vi "Generate String.vi"(8 "error in (no error)":errorcluster, 11 "object in":refnum<class "RawCodeElement.lvclass">) -> (0 "error out":errorcluster, 2 "String":string, 3 "object out":refnum<class "RawCodeElement.lvclass">)   [LabVIEW 2017, in "RawCodeElement.lvclass"]
uses:
  RawCodeElement.lvclass
  RawCodeElement.lvclass/RawCodeElement.ctl
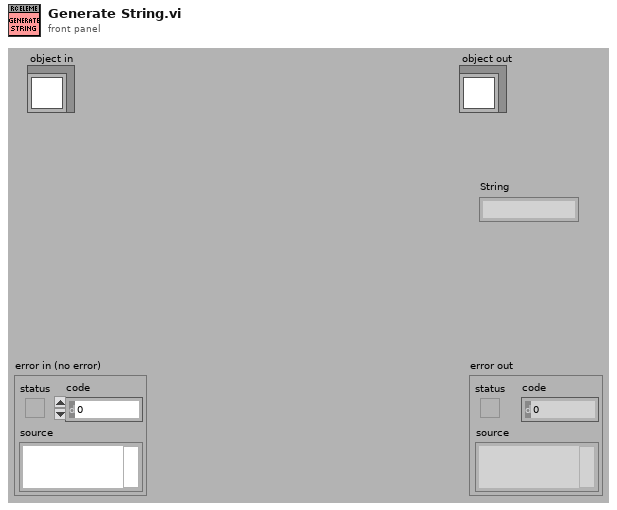
[diagram p1: front panel]
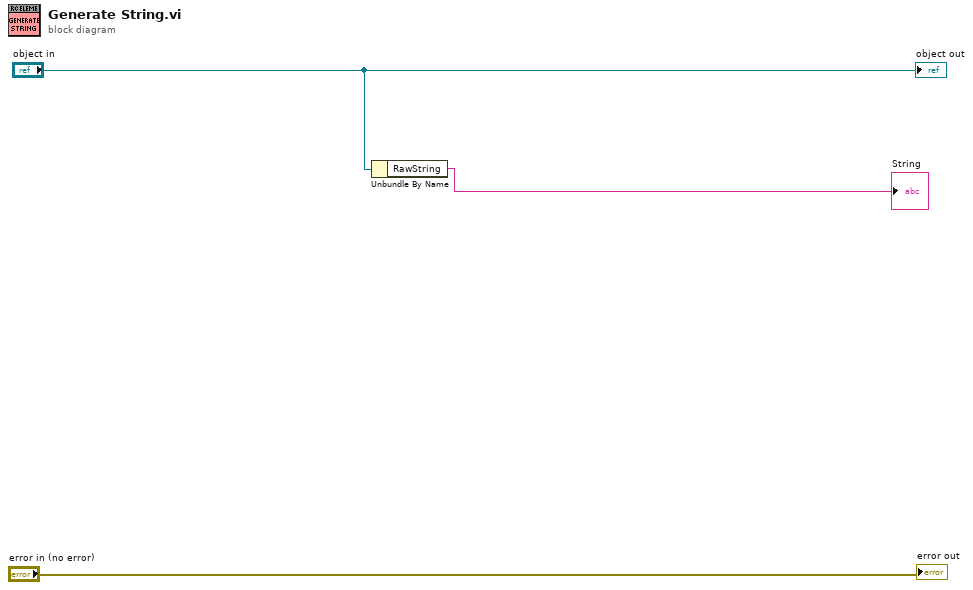
[diagram p0: block diagram]
diagram:
  n1 = Unbundle By Name("object in") -> ("RawString"=→"String":string)
  "error out" <- "error in (no error)"
  "object out" <- "object in"
